vi "Vision Processing.vi"(4 "error in (no error)":errorcluster, 7 "Image Size":T1=enum."320x240") -> ()   [LabVIEW 2015]
doc: "This VI runs in parallel to other tasks. It gets images from the camera, processes them for color or shape and use that information to affect robot behavior."
uses:
  <vilib>/Rock Robotics/WPI/Camera/WPI_CameraImageSize.ctl
  <vilib>/Rock Robotics/WPI/Camera/WPI_CameraWhite Balance Values.ctl
  <vilib>/Rock Robotics/WPI/Camera/WPI_CameraExposure Values.ctl
  <vilib>/Rock Robotics/WPI/Camera/WPI_CameraFrameRate.ctl
  Robot Global Data.vi
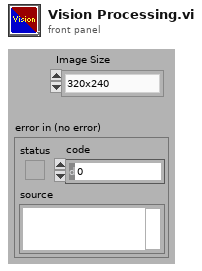
[diagram p1: front panel]
types:
  T1 = typedef "WPI_CameraImageSize.ctl" = enum16{"640x480", "320x240", "160x120", "Custom"}
  T2 = typedef "WPI_CameraFrameRate.ctl" = u32
  T3 = typedef "WPI_CameraExposure Values.ctl" = enum16{"Auto", "Flicker-free 50 Hz", "Flicker-free 60 Hz", "Hold current", "Custom"}
  T4 = typedef "WPI_CameraWhite Balance Values.ctl" = enum16{"Auto", "Fixed indoor", "Fixed outdoor 1", "Fixed outdoor 2", "Fixed fluorescent 1", "Fixed fluorescent 2", "Hold current", "Custom"}
  T5 = typedef "Image Type" = u32
  T6 = typedef "WPI_CameraDevRef.ctl" = cluster{"Camera Address":string, "CameraStatus":errorcluster}
  T7 = typedef "IMAQ Image.ctl" = refnum<image>
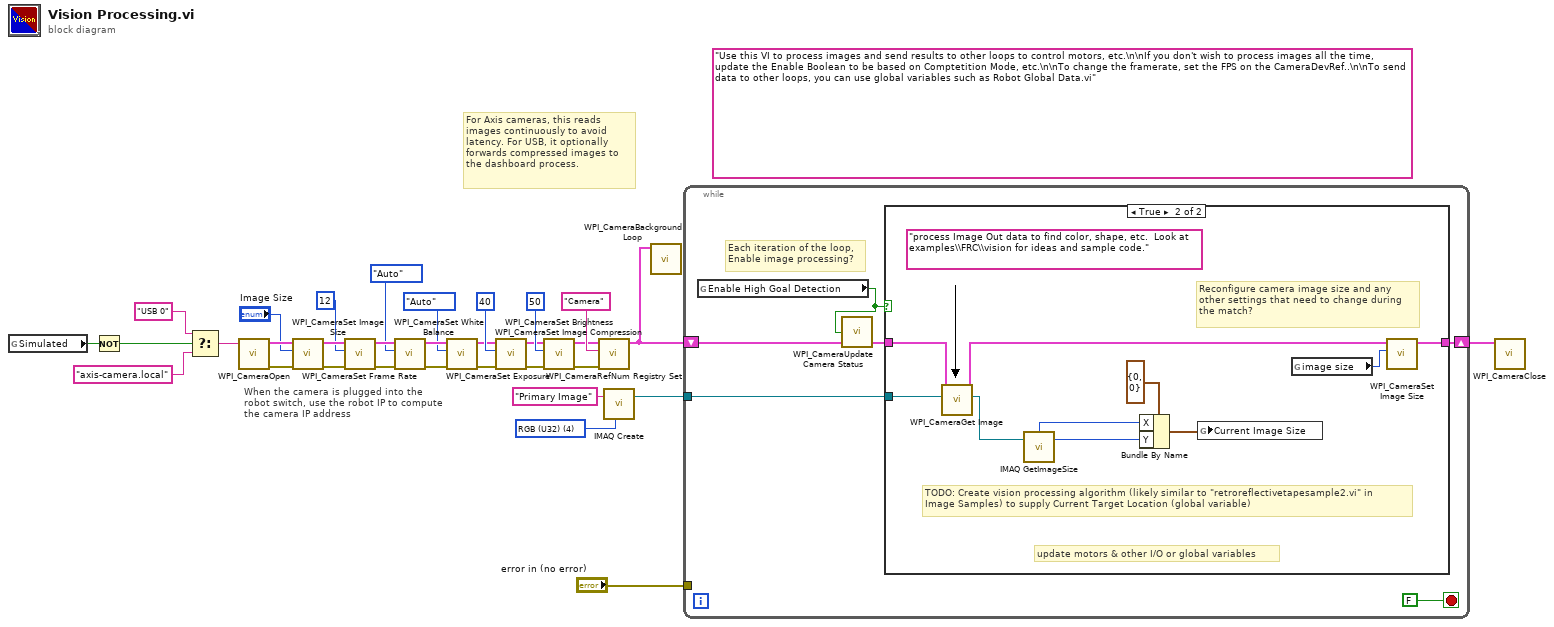
[diagram p0: block diagram]
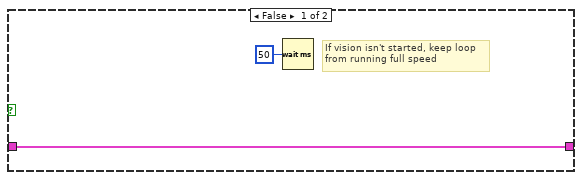
[diagram p2: hidden frame]
diagram:
  (unwired) "Use this VI to process images and send results to other loops to control motors, etc.\n\nIf you don't wish to process images all the time, update the Enable Boolean to be based on Comptetition Mode, etc.\n\nTo change the framerate, set the FPS on the CameraDevRef..\n\nTo send data to other loops, you can use global variables such as Robot Global Data.vi"
  w32 = T5 4 items=["Grayscale (U8)", "Grayscale (I16)", "Grayscale (SGL)", "Complex (CSG)", "RGB (U32)", "HSL (U32)", "RGB (U64)"] ("Image Type")
  # "When the camera is plugged into the\nrobot switch, use the robot IP to compute\nthe camera IP address"
  # "For Axis cameras, this reads\nimages continuously to avoid\nlatency. For USB, it optionally\nforwards compressed images to\nthe dashboard process."
  n1 = global read "Robot Global Data.vi" "Simulated"() -> (w2:bool)
  n2 = Not(x=w2) -> (.not. x?=w1:bool)
  n3 = Select(t="USB 0" ("format string"), s=w1, f="axis-camera.local" ("format string")) -> (s? t:f=w4:string)
  n4 = call <vilib>:"WPI_CameraOpen.vi"("Camera Address"=w4) -> ("error out"=w20:errorcluster, "CameraDevRef"=w21:T6)  [unwired: 2 in, 7 out]
  n5 = call <vilib>:"WPI_CameraSet Image Size.vi"("error in (no error)"=w20, "Image Size"="Image Size", "CameraDevRef"=w21) -> ("error out"=w19:errorcluster, "CameraDevRef Out"=w22:T6)  [unwired: 1 in, 6 out]
  n6 = call <vilib>:"WPI_CameraSet Frame Rate.vi"("error in (no error)"=w19, "Frame Rate (fps)"=T2 12, "CameraDevRef"=w22) -> ("error out"=w18:errorcluster, "CameraDevRef Out"=w24:T6)  [unwired: 7 out]
  n7 = call <vilib>:"WPI_CameraSet White Balance.vi"("error in (no error)"=w18, "White Balance"=WPI_CameraWhite_Balance_Values."Auto", "CameraDevRef"=w24) -> ("error out"=w17:errorcluster, "CameraDevRef Out"=w23:T6)  [unwired: 1 in, 6 out]
  n8 = call <vilib>:"WPI_CameraSet Exposure.vi"("error in (no error)"=w17, "Exposure"=WPI_CameraExposure_Values."Auto", "CameraDevRef"=w23) -> ("error out"=w16:errorcluster, "CameraDevRef Out"=w26:T6)  [unwired: 1 in, 6 out]
  n9 = call <vilib>:"WPI_CameraSet Image Compression.vi"("error in (no error)"=w16, "Compression"=40, "CameraDevRef"=w26) -> ("error out"=w15:errorcluster, "CameraDevRef Out"=w25:T6)  [unwired: 7 out]
  n10 = call <vilib>:"WPI_CameraSet Brightness.vi"("error in (no error)"=w15, "Brightness"=50, "CameraDevRef"=w25) -> ("error out"=w13:errorcluster, "CameraDevRef Out"=w14:T6)  [unwired: 7 out]
  n11 = call <vilib>:"WPI_CameraRefNum Registry Set.vi"("error in (no error)"=w13, "refnum name"="Camera", "CameraDevRef"=w14) -> ("CameraDevRef"=w9:T6)  [unwired: 1 in, 7 out]
  n12 = call "IMAQ Create"("Image Name"="Primary Image", "Image Type"=w32) -> ("New Image"=w30:T7)  [unwired: 2 in, 2 out]
  n13 = call <vilib>:"WPI_CameraBackground Loop.vi"("CameraDevRef"=w9) -> ()  [unwired: 11 in]
  n14 = while {
    shift-right: [w37] -> w7
    shift-left: w9 -> [w35]
    tunnel: w30 -> [w36]
    tunnel: "error in (no error)" -> [_]
    stop <- FALSE stop-if-true
    # "Each iteration of the loop,\nEnable image processing?"
    n15 = global read "Robot Global Data.vi" "Enable High Goal Detection"() -> (w33:bool)
    n16 = call <vilib>:"WPI_CameraUpdate Camera Status.vi"("CameraDevRef In"=w35, "Enable Vision"=w33) -> ("CameraDevRef Out"=w34:T6)  [unwired: 3 in]
    n17 = case shown="True" w33 {
      tunnel: w36 -> [_ w49]
      tunnel: [w40 w50] -> w37
      tunnel: w34 -> [w40 w47]
      frame False {
        # "If vision isn't started, keep loop\nfrom running full speed"
        n18 = Wait (ms)(milliseconds to wait=u32 50) -> ()  [unwired: 1 out]
      }
      frame True {
        (unwired) "process Image Out data to find color, shape, etc.  Look at examples\\FRC\\vision for ideas and sample code."
        # "TODO: Create vision processing algorithm (likely similar to \"retroreflectivetapesample2.vi\" in\nImage Samples) to supply Current Target Location (global variable)"
        # "update motors & other I/O or global variables"
        # "Reconfigure camera image size and any\nother settings that need to change during\nthe match?"
        n19 = call <vilib>:"WPI_CameraGet Image.vi"("Image"=w49, "CameraDevRef"=w47) -> ("Image Out"=w45:T7, "CameraDevRef Out"=w46:T6)  [unwired: 1 in, 7 out]
        n20 = call "IMAQ GetImageSize"("Image"=w45) -> ("Y Resolution"=w42:i32, "X Resolution"=w43:i32)  [unwired: 3 in, 1 out]
        n21 = Bundle By Name(cluster=cluster{"X":i32, "Y":i32} {"X"=0, "Y"=0} ("Current Image Size"), "X"=w43, "Y"=w42) -> (w41:cluster{"X":i32, "Y":i32})
        n22 = global write "Robot Global Data.vi" "Current Image Size"(w41) -> ()
        n23 = global read "Robot Global Data.vi" "image size"() -> (w48:T1)
        n24 = call <vilib>:"WPI_CameraSet Image Size.vi"("Image Size"=w48, "CameraDevRef"=w46) -> ("CameraDevRef Out"=w50:T6)  [unwired: 2 in, 7 out]
      }
    }
  }
  n25 = call <vilib>:"WPI_CameraClose.vi"("CameraDevRef"=w7) -> ()  [unwired: 1 in, 10 out]
